vi "TCP-Get Subnet Address.vi"(7 "net address":u32) -> (8 "subnet address":u32, 10 "subnet address":string)   [LabVIEW 2020]
uses:
  <vilib>/regexp/Match Regular Expression.xnode
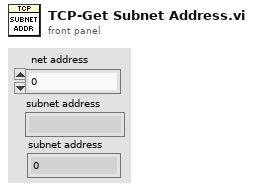
[diagram p1: front panel]
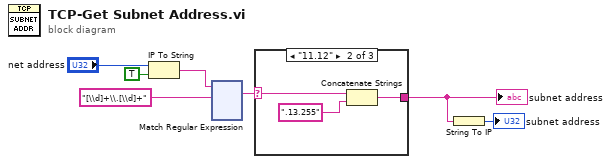
[diagram p0: block diagram]
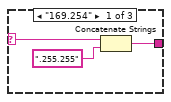
[diagram p2: hidden frame]
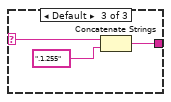
[diagram p3: hidden frame]
diagram:
  n1 = IP To String(1:TRUE ("dot notation? (F)"), 2:"net address") -> (0:w3:string)
  n2 = xnode "Match Regular Expression"("input string"=w3, "regular expression"="[\\d]+\\.[\\d]+") -> ("whole match"=w4:string)  [unwired: 4 in, 4 out]
  n3 = case shown="\"11.12\"" w4 {
    selector: w4 -> [w10 w13 w16]
    tunnel: [w8 w11 w14] -> w1
    frame "169.254" {
      n4 = Concatenate Strings(w10, ".255.255") -> (w8:string)
    }
    frame "11.12" {
      n5 = Concatenate Strings(w13, ".13.255") -> (w11:string)
    }
    frame Default {
      n6 = Concatenate Strings(w16, ".1.255") -> (w14:string)
    }
  }
  "subnet address" <- w1
  n7 = String To IP(1:w1) -> (0:→"subnet address":u32)
